vi "Insert Panel To Controller.vi"(0 "Microscope Controller in":refnum<class "Microscope Controller.lvclass">, 5 "Sub Panel":string, 9 "VI Refnum":refnum<vi>, 11 "error in (no error)":errorcluster) -> (4 "Microscope Controller out":refnum<class "Microscope Controller.lvclass">, 15 "error out":errorcluster)   [LabVIEW 2020]
uses:
  Microscope Controller.lvclass
  C:/Program Files/National Instruments/LabVIEW 2020/vi.lib/ActorFramework/Actor/Actor.lvclass
  E:/Development/DevHardSoftware/MicroscopyFramework/ViewController/Microscope Controller/Microscope Controller.lvclass
  E:/Development/DevHardSoftware/MicroscopyFramework/MicroscopeControllerIO/MicroscopeControllerIO.lvclass
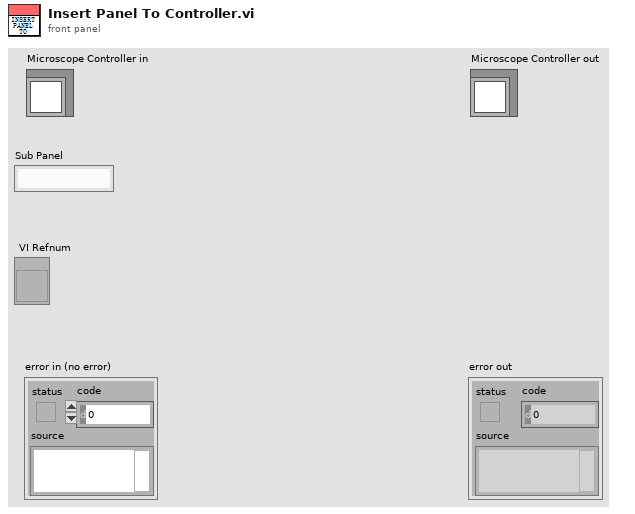
[diagram p1: front panel]
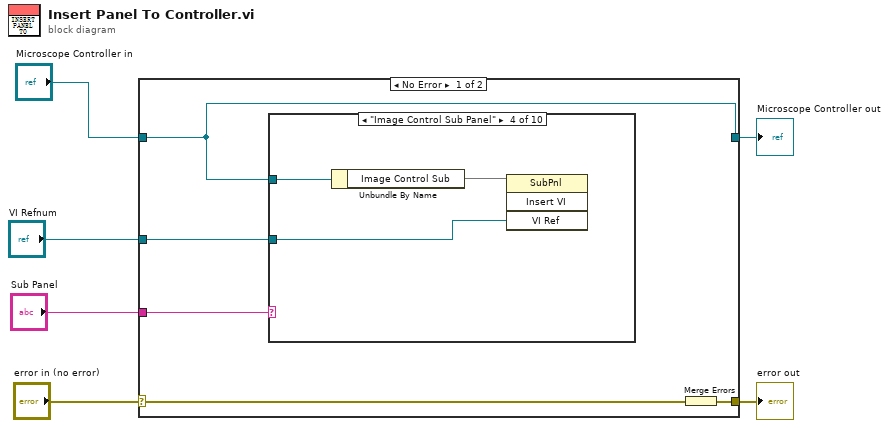
[diagram p0: block diagram]
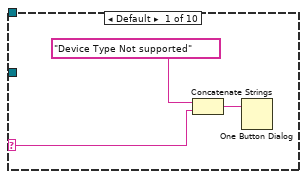
[diagram p2: hidden frame]
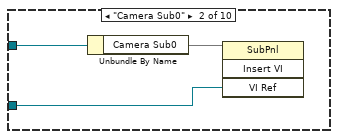
[diagram p3: hidden frame]
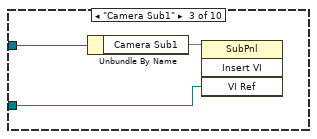
[diagram p4: hidden frame]
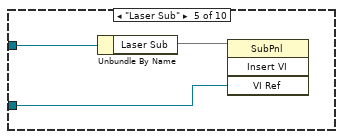
[diagram p5: hidden frame]
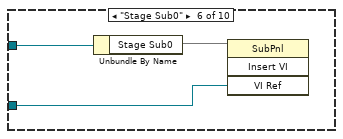
[diagram p6: hidden frame]
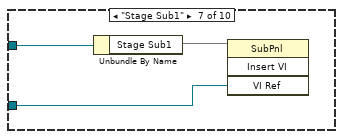
[diagram p7: hidden frame]
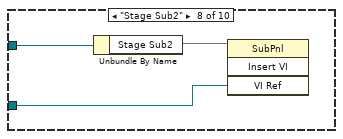
[diagram p8: hidden frame]
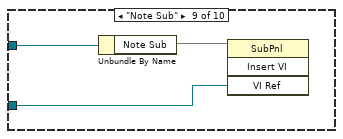
[diagram p9: hidden frame]
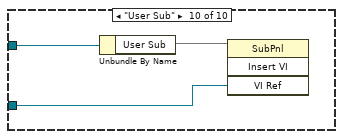
[diagram p10: hidden frame]
diagram:
  n1 = case shown="No Error" "error in (no error)" {
    selector: "error in (no error)" -> [w10 w43]
    tunnel: [w9 w43] -> w5
    tunnel: [w11 w42] -> w3
    tunnel: "Microscope Controller in" -> [w11 w42]
    tunnel: "VI Refnum" -> [w8 _]
    tunnel: "Sub Panel" -> [w7 _]
    frame No Error {
      n2 = case shown="\"Image Control Sub Panel\"" w7 {
        selector: w7 -> [w13 _ _ _ _ _ _ _ _ _]
        tunnel: w11 -> [_ w17 w20 w23 w26 w29 w32 w35 w38 w41]
        tunnel: w8 -> [_ w15 w18 w21 w24 w27 w30 w33 w36 w39]
        frame Default {
          n3 = Concatenate Strings("Device Type Not supported" ("string"), w13) -> (w14:string)
          n4 = One Button Dialog(message=w14) -> ()  [unwired: 1 in, 1 out]
        }
        frame "Camera Sub0" {
          n5 = Unbundle By Name(w17) -> ("Camera Sub0"=w16)
          n6 = invoke class="SubPnl" method="Insert VI"(reference=w16, "VI Ref"=w15) -> ()  [unwired: 2 in, 4 out]
        }
        frame "Camera Sub1" {
          n7 = Unbundle By Name(w20) -> ("Camera Sub1"=w19)
          n8 = invoke class="SubPnl" method="Insert VI"(reference=w19, "VI Ref"=w18) -> ()  [unwired: 2 in, 4 out]
        }
        frame "Image Control Sub Panel" {
          n9 = Unbundle By Name(w23) -> ("Image Control Sub"=w22)
          n10 = invoke class="SubPnl" method="Insert VI"(reference=w22, "VI Ref"=w21) -> ()  [unwired: 2 in, 4 out]
        }
        frame "Laser Sub" {
          n11 = Unbundle By Name(w26) -> ("Laser Sub"=w25)
          n12 = invoke class="SubPnl" method="Insert VI"(reference=w25, "VI Ref"=w24) -> ()  [unwired: 2 in, 4 out]
        }
        frame "Stage Sub0" {
          n13 = Unbundle By Name(w29) -> ("Stage Sub0"=w28)
          n14 = invoke class="SubPnl" method="Insert VI"(reference=w28, "VI Ref"=w27) -> ()  [unwired: 2 in, 4 out]
        }
        frame "Stage Sub1" {
          n15 = Unbundle By Name(w32) -> ("Stage Sub1"=w31)
          n16 = invoke class="SubPnl" method="Insert VI"(reference=w31, "VI Ref"=w30) -> ()  [unwired: 2 in, 4 out]
        }
        frame "Stage Sub2" {
          n17 = Unbundle By Name(w35) -> ("Stage Sub2"=w34)
          n18 = invoke class="SubPnl" method="Insert VI"(reference=w34, "VI Ref"=w33) -> ()  [unwired: 2 in, 4 out]
        }
        frame "Note Sub" {
          n19 = Unbundle By Name(w38) -> ("Note Sub"=w37)
          n20 = invoke class="SubPnl" method="Insert VI"(reference=w37, "VI Ref"=w36) -> ()  [unwired: 2 in, 4 out]
        }
        frame "User Sub" {
          n21 = Unbundle By Name(w41) -> ("User Sub"=w40)
          n22 = invoke class="SubPnl" method="Insert VI"(reference=w40, "VI Ref"=w39) -> ()  [unwired: 2 in, 4 out]
        }
      }
      n23 = Merge Errors(w10) -> (w9:errorcluster)
    }
    frame Error {
    }
  }
  "error out" <- w5
  "Microscope Controller out" <- w3
